vi "simple write tdms.vi"() -> ()   [LabVIEW 2022 SP3]
panel:
  in  "channel name(s) in (Untitled)":string[](array[string])
  in  "group name in (Untitled)":string
  in  "file path":path
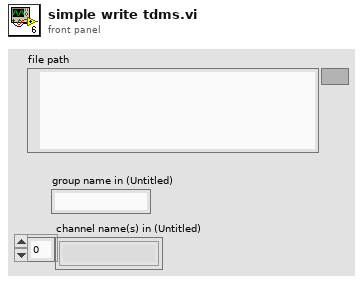
[diagram p1: front panel]
types:
  T1 = enum16{"open", "open or create", "create or replace", "create", "open (read-only)"}
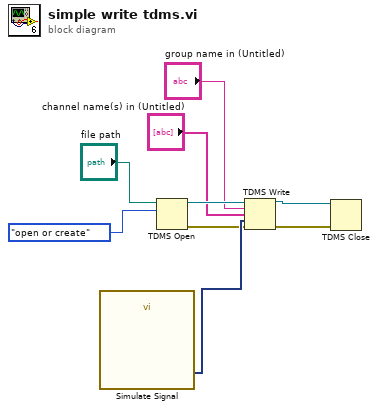
[diagram p0: block diagram]
diagram:
  n1 = call "Simulate Signal"() -> ("Sine"=w4:dynamicdata)  [unwired: 14 in, 1 out]
  n2 = TDMS Open(10:T1."open or create" ("operation (0:open)"), 11:"file path") -> (0:w1:errorcluster, 3:w7:refnum<k34>)  [unwired: 5 in]
  n3 = TDMS Write(0:w7, 5:"group name in (Untitled)", 7:"channel name(s) in (Untitled)", 9:w4, 11:w1) -> (4:w3:refnum<k34>, 15:w2:errorcluster)  [unwired: 1 in, 2 out]
  n4 = TDMS Close(8:w2, 11:w3) -> ()  [unwired: 2 out]
